vi "about get DF index details.vi"(8 "error in (no error)":errorcluster) -> (0 "error out":errorcluster, 3 "Index Details":T1, 5 "Data Repository Path":path)   [LabVIEW 2011]
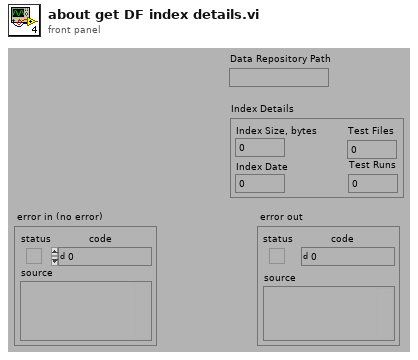
[diagram p1: front panel]
types:
  T1 = cluster{"Index Size, bytes":i64, "Index Date":dbl, "Test Files":i32, "Test Runs":i32}
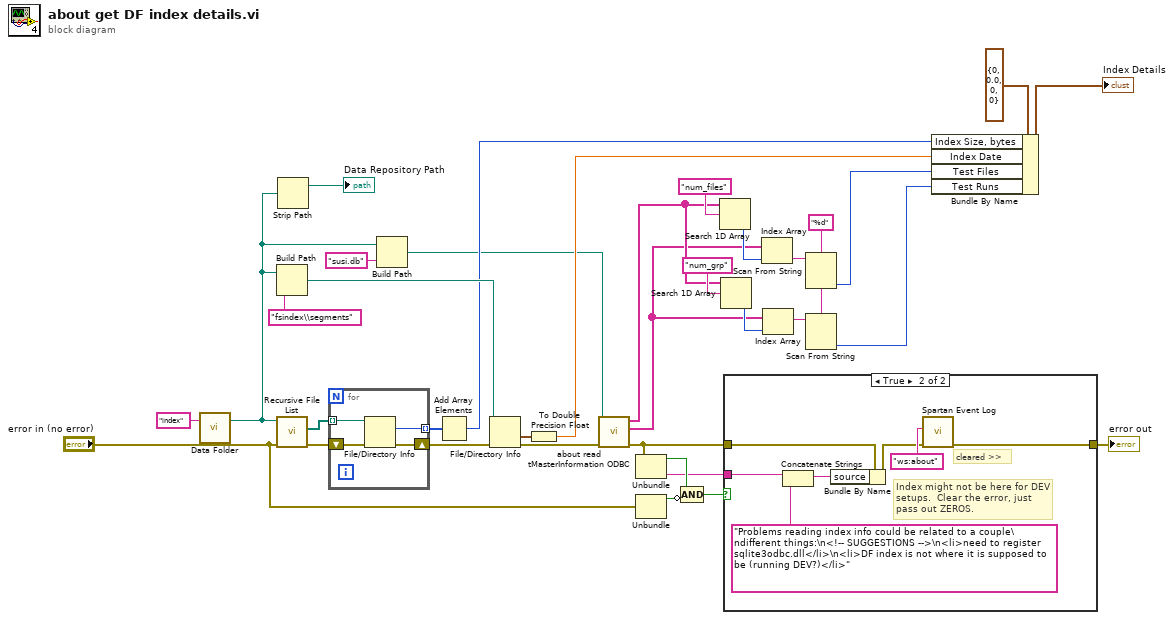
[diagram p0: block diagram]
diagram:
  w15 = "%d"
  n1 = call "Data Folder.vi"("Relative Path (\"\" - Folder)"="index" ("Relative Path (\"\" - Folder)")) -> ("Data Folder"=w2:path)  [unwired: 2 in]
  n2 = Build Path(base path=w2, name or relative path="fsindex\\segments" ("Relative Path (\"\" - Folder)")) -> (appended path=w28:path)
  n3 = call <vilib>:"Recursive File List.vi"("error in (no error)"="error in (no error)", "Folder Path"=w2) -> ("error out"=w32:errorcluster, "All Files in Dir"=w34:path[])  [unwired: 1 in, 7 out]
  n4 = Strip Path(path=w2) -> (stripped path=→"Data Repository Path":path)  [unwired: 1 out]
  n5 = for {
    tunnel: w34 -> [w39] mode=indexing
    tunnel: [w38] -> w33 mode=indexing
    shift-right: [w36] -> w25
    shift-left: w32 -> [w37]
    n6 = File/Directory Info(path=w39, error in=w37) -> (size=w38:i64, error out=w36:errorcluster)  [unwired: 5 out]
  }
  n7 = Build Path(base path=w2, name or relative path="susi.db") -> (appended path=w12:path)
  n8 = Add Array Elements(numeric array=w33) -> (sum=w26:i64)
  n9 = File/Directory Info(path=w28, error in=w25) -> (last mod=w30:timestamp, error out=w13:errorcluster)  [unwired: 5 out]
  n10 = To Double Precision Float(number=w30) -> (double precision float=w24:dbl)
  n11 = call "about read tMasterInformation ODBC.vi"("error in (no error)"=w13, "DF Index db (\"\")"=w12) -> ("error out"=w8:errorcluster, "values"=w10:string[], "names"=w11:string[])  [unwired: 1 in, 6 out]
  n12 = Unbundle(w8) -> ("status"=w6:bool, "source"=w3:string)  [unwired: 1 out]
  n13 = Unbundle("error in (no error)") -> ("status"=w5:bool)  [unwired: 2 out]
  n14 = Compound Arithmetic op=AND(w6, invert w5) -> (w4:bool)
  n15 = Search 1D Array(1D array=w11, element="num_files") -> (index of element=w21:i32)  [unwired: 1 out]
  n16 = Search 1D Array(1D array=w11, element="num_grp") -> (index of element=w20:i32)  [unwired: 1 out]
  n17 = case shown="True" w4 {
    tunnel: w8 -> [w40 w45]
    tunnel: [w40 w47] -> w9
    tunnel: w3 -> [_ w43]
    frame False {
    }
    frame True {
      # "cleared >>"
      # "Index might not be here for DEV\nsetups.  Clear the error, just\npass out ZEROS."
      n18 = Concatenate Strings(w43, "Problems reading index info could be related to a couple\ndifferent things:\n<!-- SUGGESTIONS -->\n<li>need to register sqlite3odbc.dll</li>\n<li>DF index is not where it is supposed to be (running DEV?)</li>") -> (w41:string)
      n19 = Bundle By Name(cluster=w45, "source"=w41) -> (w44:errorcluster)
      n20 = call "Spartan Event Log.vi"("error in (no error)"=w44, "module (\"\")"="ws:about") -> ("error out"=w47:errorcluster)  [unwired: 6 in]
    }
  }
  "error out" <- w9
  n21 = Index Array(array=w10, index=w21) -> (element=w18:string)
  n22 = Index Array(array=w10, index=w20) -> (element=w16:string)
  n23 = Scan From String(format string=w15, input string=w18) -> (output 1=w17:i32)  [unwired: 2 in, 4 out]
  n24 = Scan From String(format string=w15, input string=w16) -> (output 1=w14:i32)  [unwired: 2 in, 4 out]
  n25 = Bundle By Name(cluster=T1 {"Index Size, bytes"=0, "Index Date"=0.0, "Test Files"=0, "Test Runs"=0} ("Index Details"), "Index Size, bytes"=w26, "Index Date"=w24, "Test Files"=w17, "Test Runs"=w14) -> (→"Index Details":T1)
